vi "F Dwf Digital Out Wait Get.vi"(8 "error in (no error)":errorcluster, 10 "psecWait":dbl, 11 "hdwf":i32) -> (0 "error out":errorcluster, 2 "psecWait out":dbl, 3 "function return":i32)   [LabVIEW 2021, in "Olasdwf.lvlib"]
doc: "DWFAPI int FDwfDigitalOutWaitGet(HDWF hdwf, double *psecWait);"
uses:
  Olasdwf.lvlib
  Windows/System32/dwf.dll
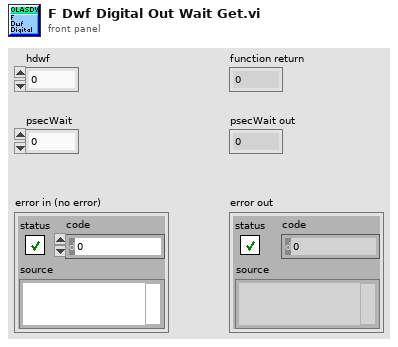
[diagram p1: front panel]
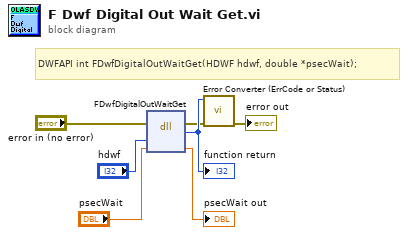
[diagram p0: block diagram]
diagram:
  # "DWFAPI int FDwfDigitalOutWaitGet(HDWF hdwf, double *psecWait);"
  n1 = dll-call lib="/Windows/System32/dwf.*" fn="FDwfDigitalOutWaitGet"(error in="error in (no error)", "hdwf"="hdwf", "psecWait"="psecWait") -> (error out=w2:errorcluster, w7:i32, "psecWait"=→"psecWait out":dbl)  [unwired: 3 in, 1 out]
  "function return" <- w7
  n2 = call "Error Converter (ErrCode or Status).vi"("error in (no error)"=w2, "error code"=w7) -> ("error out"=→"error out":errorcluster)  [unwired: 9 in]
